vi "lvpeak_interpret_status_code.vi"(10 "status_code":i32 format="%x", 11 "error in (no error)":errorcluster) -> (3 "error out":errorcluster {"code" format="%x"})   [LabVIEW 2024, in "Vision.lvlib"]
uses:
  Vision.lvlib
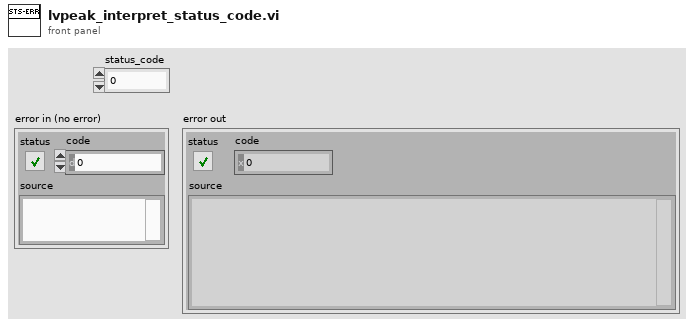
[diagram p1: front panel]
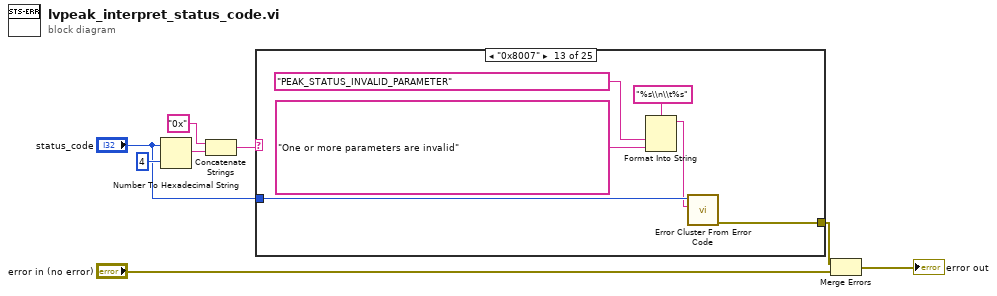
[diagram p0: block diagram]
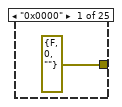
[diagram p2: hidden frame]
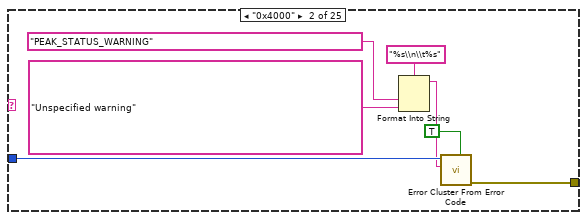
[diagram p3: hidden frame]
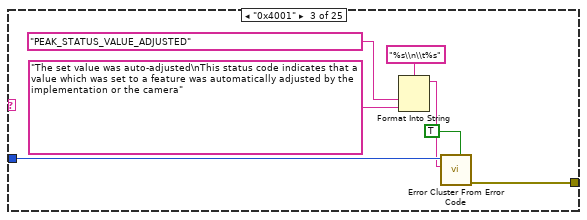
[diagram p4: hidden frame]
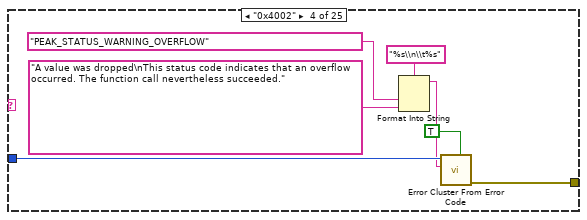
[diagram p5: hidden frame]
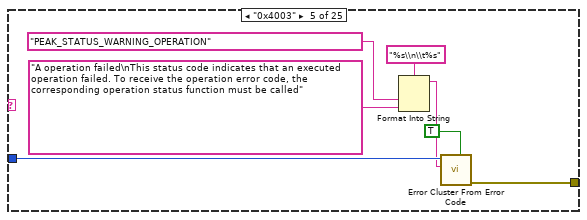
[diagram p6: hidden frame]
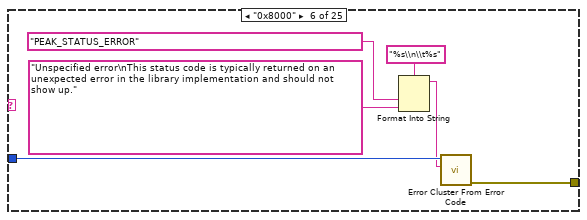
[diagram p7: hidden frame]
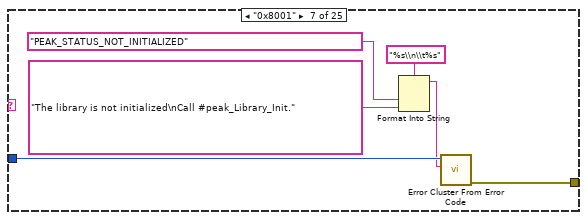
[diagram p8: hidden frame]
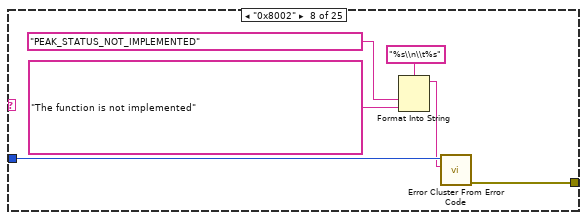
[diagram p9: hidden frame]
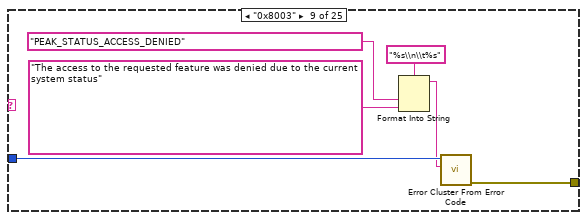
[diagram p10: hidden frame]
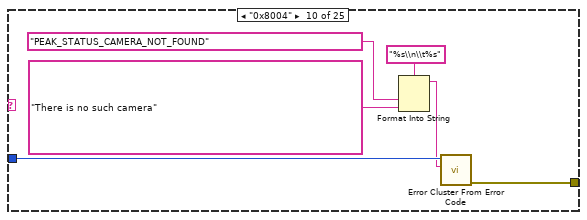
[diagram p11: hidden frame]
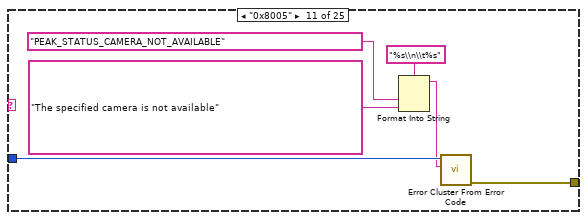
[diagram p12: hidden frame]
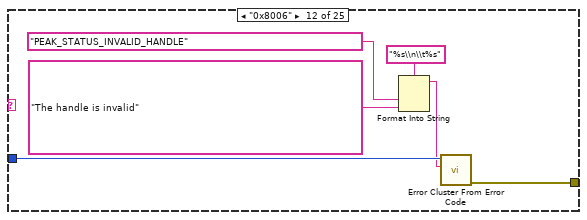
[diagram p13: hidden frame]
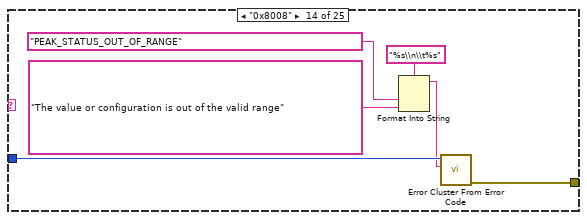
[diagram p14: hidden frame]
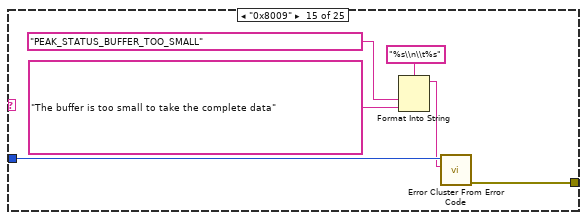
[diagram p15: hidden frame]
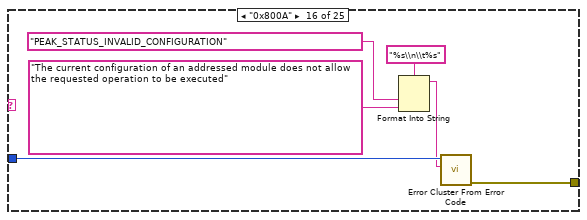
[diagram p16: hidden frame]
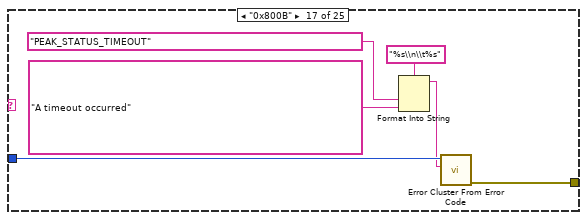
[diagram p17: hidden frame]
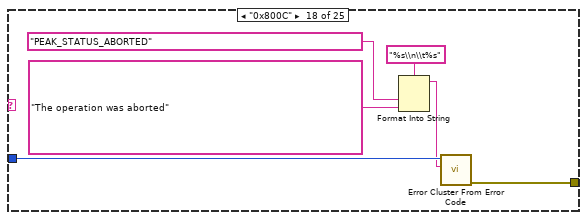
[diagram p18: hidden frame]
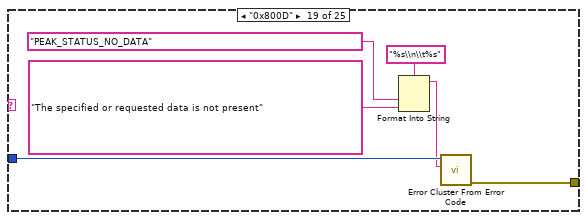
[diagram p19: hidden frame]
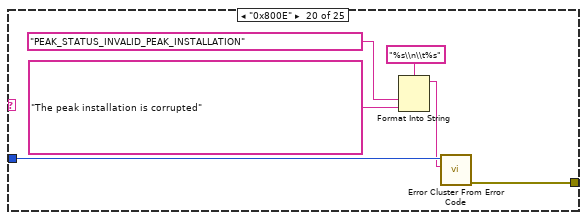
[diagram p20: hidden frame]
diagram:
  n1 = Number To Hexadecimal String(1:i16 4 ("width (-)"), 2:"status_code") -> (0:w7:string)
  n2 = Concatenate Strings("0x" ("string"), w7) -> (w5:string)
  n3 = case shown="\"0x8007\"" w5 {
    tunnel: "status_code" -> [_ w16 w23 w30 w37 w43 w49 w55 w61 w67 w73 w79 w85 w91 w97 w103 w109 w115 w121 w127 w133 w139 w145 w151 w152]
    tunnel: [errorcluster {"status"=FALSE, "code"=0, "source"=""} ("error out") w15 w22 w29 w36 w42 w48 w54 w60 w66 w72 w78 w84 w90 w96 w102 w108 w114 w120 w126 w132 w138 w144 w150 w156] -> w3
    frame "0x0000" {
    }
    frame "0x4000" {
      n4 = Format Into String(format string="%s\\n\\t%s", "PEAK_STATUS_WARNING", "Unspecified warning") -> (resulting string=w11:string)  [unwired: 2 in, 1 out]
      n5 = call <vilib>:"Error Cluster From Error Code.vi"("is warning? (False)"=TRUE, "error message (\"\")"=w11, "error code (0)"=w16) -> ("error out"=w15:errorcluster)  [unwired: 6 in]
    }
    frame "0x4001" {
      n6 = Format Into String(format string="%s\\n\\t%s", "PEAK_STATUS_VALUE_ADJUSTED", "The set value was auto-adjusted\nThis status code indicates that a value which was set to a feature was automatically adjusted by the implementation or the camera") -> (resulting string=w18:string)  [unwired: 2 in, 1 out]
      n7 = call <vilib>:"Error Cluster From Error Code.vi"("is warning? (False)"=TRUE, "error message (\"\")"=w18, "error code (0)"=w23) -> ("error out"=w22:errorcluster)  [unwired: 6 in]
    }
    frame "0x4002" {
      n8 = Format Into String(format string="%s\\n\\t%s", "PEAK_STATUS_WARNING_OVERFLOW", "A value was dropped\nThis status code indicates that an overflow occurred. The function call nevertheless succeeded.") -> (resulting string=w25:string)  [unwired: 2 in, 1 out]
      n9 = call <vilib>:"Error Cluster From Error Code.vi"("is warning? (False)"=TRUE, "error message (\"\")"=w25, "error code (0)"=w30) -> ("error out"=w29:errorcluster)  [unwired: 6 in]
    }
    frame "0x4003" {
      n10 = Format Into String(format string="%s\\n\\t%s", "PEAK_STATUS_WARNING_OPERATION", "A operation failed\nThis status code indicates that an executed operation failed. To receive the operation error code, the corresponding operation status function must be called") -> (resulting string=w32:string)  [unwired: 2 in, 1 out]
      n11 = call <vilib>:"Error Cluster From Error Code.vi"("is warning? (False)"=TRUE, "error message (\"\")"=w32, "error code (0)"=w37) -> ("error out"=w36:errorcluster)  [unwired: 6 in]
    }
    frame "0x8000" {
      n12 = Format Into String(format string="%s\\n\\t%s", "PEAK_STATUS_ERROR", "Unspecified error\nThis status code is typically returned on an unexpected error in the library implementation and should not show up.") -> (resulting string=w38:string)  [unwired: 2 in, 1 out]
      n13 = call <vilib>:"Error Cluster From Error Code.vi"("error message (\"\")"=w38, "error code (0)"=w43) -> ("error out"=w42:errorcluster)  [unwired: 7 in]
    }
    frame "0x8001" {
      n14 = Format Into String(format string="%s\\n\\t%s", "PEAK_STATUS_NOT_INITIALIZED", "The library is not initialized\nCall #peak_Library_Init.") -> (resulting string=w44:string)  [unwired: 2 in, 1 out]
      n15 = call <vilib>:"Error Cluster From Error Code.vi"("error message (\"\")"=w44, "error code (0)"=w49) -> ("error out"=w48:errorcluster)  [unwired: 7 in]
    }
    frame "0x8002" {
      n16 = Format Into String(format string="%s\\n\\t%s", "PEAK_STATUS_NOT_IMPLEMENTED", "The function is not implemented") -> (resulting string=w50:string)  [unwired: 2 in, 1 out]
      n17 = call <vilib>:"Error Cluster From Error Code.vi"("error message (\"\")"=w50, "error code (0)"=w55) -> ("error out"=w54:errorcluster)  [unwired: 7 in]
    }
    frame "0x8003" {
      n18 = Format Into String(format string="%s\\n\\t%s", "PEAK_STATUS_ACCESS_DENIED", "The access to the requested feature was denied due to the current system status") -> (resulting string=w56:string)  [unwired: 2 in, 1 out]
      n19 = call <vilib>:"Error Cluster From Error Code.vi"("error message (\"\")"=w56, "error code (0)"=w61) -> ("error out"=w60:errorcluster)  [unwired: 7 in]
    }
    frame "0x8004" {
      n20 = Format Into String(format string="%s\\n\\t%s", "PEAK_STATUS_CAMERA_NOT_FOUND", "There is no such camera") -> (resulting string=w62:string)  [unwired: 2 in, 1 out]
      n21 = call <vilib>:"Error Cluster From Error Code.vi"("error message (\"\")"=w62, "error code (0)"=w67) -> ("error out"=w66:errorcluster)  [unwired: 7 in]
    }
    frame "0x8005" {
      n22 = Format Into String(format string="%s\\n\\t%s", "PEAK_STATUS_CAMERA_NOT_AVAILABLE", "The specified camera is not available") -> (resulting string=w68:string)  [unwired: 2 in, 1 out]
      n23 = call <vilib>:"Error Cluster From Error Code.vi"("error message (\"\")"=w68, "error code (0)"=w73) -> ("error out"=w72:errorcluster)  [unwired: 7 in]
    }
    frame "0x8006" {
      n24 = Format Into String(format string="%s\\n\\t%s", "PEAK_STATUS_INVALID_HANDLE", "The handle is invalid") -> (resulting string=w74:string)  [unwired: 2 in, 1 out]
      n25 = call <vilib>:"Error Cluster From Error Code.vi"("error message (\"\")"=w74, "error code (0)"=w79) -> ("error out"=w78:errorcluster)  [unwired: 7 in]
    }
    frame "0x8007" {
      n26 = Format Into String(format string="%s\\n\\t%s", "PEAK_STATUS_INVALID_PARAMETER", "One or more parameters are invalid") -> (resulting string=w80:string)  [unwired: 2 in, 1 out]
      n27 = call <vilib>:"Error Cluster From Error Code.vi"("error message (\"\")"=w80, "error code (0)"=w85) -> ("error out"=w84:errorcluster)  [unwired: 7 in]
    }
    frame "0x8008" {
      n28 = Format Into String(format string="%s\\n\\t%s", "PEAK_STATUS_OUT_OF_RANGE", "The value or configuration is out of the valid range") -> (resulting string=w86:string)  [unwired: 2 in, 1 out]
      n29 = call <vilib>:"Error Cluster From Error Code.vi"("error message (\"\")"=w86, "error code (0)"=w91) -> ("error out"=w90:errorcluster)  [unwired: 7 in]
    }
    frame "0x8009" {
      n30 = Format Into String(format string="%s\\n\\t%s", "PEAK_STATUS_BUFFER_TOO_SMALL", "The buffer is too small to take the complete data") -> (resulting string=w92:string)  [unwired: 2 in, 1 out]
      n31 = call <vilib>:"Error Cluster From Error Code.vi"("error message (\"\")"=w92, "error code (0)"=w97) -> ("error out"=w96:errorcluster)  [unwired: 7 in]
    }
    frame "0x800A" {
      n32 = Format Into String(format string="%s\\n\\t%s", "PEAK_STATUS_INVALID_CONFIGURATION", "The current configuration of an addressed module does not allow the requested operation to be executed") -> (resulting string=w98:string)  [unwired: 2 in, 1 out]
      n33 = call <vilib>:"Error Cluster From Error Code.vi"("error message (\"\")"=w98, "error code (0)"=w103) -> ("error out"=w102:errorcluster)  [unwired: 7 in]
    }
    frame "0x800B" {
      n34 = Format Into String(format string="%s\\n\\t%s", "PEAK_STATUS_TIMEOUT", "A timeout occurred") -> (resulting string=w104:string)  [unwired: 2 in, 1 out]
      n35 = call <vilib>:"Error Cluster From Error Code.vi"("error message (\"\")"=w104, "error code (0)"=w109) -> ("error out"=w108:errorcluster)  [unwired: 7 in]
    }
    frame "0x800C" {
      n36 = Format Into String(format string="%s\\n\\t%s", "PEAK_STATUS_ABORTED", "The operation was aborted") -> (resulting string=w110:string)  [unwired: 2 in, 1 out]
      n37 = call <vilib>:"Error Cluster From Error Code.vi"("error message (\"\")"=w110, "error code (0)"=w115) -> ("error out"=w114:errorcluster)  [unwired: 7 in]
    }
    frame "0x800D" {
      n38 = Format Into String(format string="%s\\n\\t%s", "PEAK_STATUS_NO_DATA", "The specified or requested data is not present") -> (resulting string=w116:string)  [unwired: 2 in, 1 out]
      n39 = call <vilib>:"Error Cluster From Error Code.vi"("error message (\"\")"=w116, "error code (0)"=w121) -> ("error out"=w120:errorcluster)  [unwired: 7 in]
    }
    frame "0x800E" {
      n40 = Format Into String(format string="%s\\n\\t%s", "PEAK_STATUS_INVALID_PEAK_INSTALLATION", "The peak installation is corrupted") -> (resulting string=w122:string)  [unwired: 2 in, 1 out]
      n41 = call <vilib>:"Error Cluster From Error Code.vi"("error message (\"\")"=w122, "error code (0)"=w127) -> ("error out"=w126:errorcluster)  [unwired: 7 in]
    }
    frame "0x800F" {
      n42 = Format Into String(format string="%s\\n\\t%s", "PEAK_STATUS_BUSY", "Device or resource is busy") -> (resulting string=w128:string)  [unwired: 2 in, 1 out]
      n43 = call <vilib>:"Error Cluster From Error Code.vi"("error message (\"\")"=w128, "error code (0)"=w133) -> ("error out"=w132:errorcluster)  [unwired: 7 in]
    }
    frame "0x8010" {
      n44 = Format Into String(format string="%s\\n\\t%s", "PEAK_STATUS_OUT_OF_MEMORY", "The system could not provide enough memory") -> (resulting string=w134:string)  [unwired: 2 in, 1 out]
      n45 = call <vilib>:"Error Cluster From Error Code.vi"("error message (\"\")"=w134, "error code (0)"=w139) -> ("error out"=w138:errorcluster)  [unwired: 7 in]
    }
    frame "0x8011" {
      n46 = Format Into String(format string="%s\\n\\t%s", "PEAK_STATUS_IO", "An I/O error occurred") -> (resulting string=w140:string)  [unwired: 2 in, 1 out]
      n47 = call <vilib>:"Error Cluster From Error Code.vi"("error message (\"\")"=w140, "error code (0)"=w145) -> ("error out"=w144:errorcluster)  [unwired: 7 in]
    }
    frame "0x8012" {
      n48 = Format Into String(format string="%s\\n\\t%s", "PEAK_STATUS_NOT_SUPPORTED", "Indicates that the requested functionality is not supported") -> (resulting string=w146:string)  [unwired: 2 in, 1 out]
      n49 = call <vilib>:"Error Cluster From Error Code.vi"("error message (\"\")"=w146, "error code (0)"=w151) -> ("error out"=w150:errorcluster)  [unwired: 7 in]
    }
    frame Default {
      n50 = Format Into String(format string="%s\\n\\tUnknown Peak status code 0x%04X", "PEAK_STATUS_UNKNOWN", w152) -> (resulting string=w153:string)  [unwired: 2 in, 1 out]
      n51 = call <vilib>:"Error Cluster From Error Code.vi"("error message (\"\")"=w153, "error code (0)"=w152) -> ("error out"=w156:errorcluster)  [unwired: 7 in]
    }
  }
  n52 = Merge Errors(w3, "error in (no error)") -> (→"error out":errorcluster)
